vi "Положение лазера (SubVI).vi"(1 "Мишень reference":refnum<vi>, 3 "XY лазера reference":refnum<vi>, 5 "Текущ. инфо reference":refnum<vi>, 11 "error in":errorcluster, 12 "X коорд.":u16, 13 "Y коорд.":u16) -> (24 "error out":errorcluster)   [LabVIEW 2013]
doc: "Изменение положения точки текущего положения лазера и кол-ва выстрелов в точку на мишени"
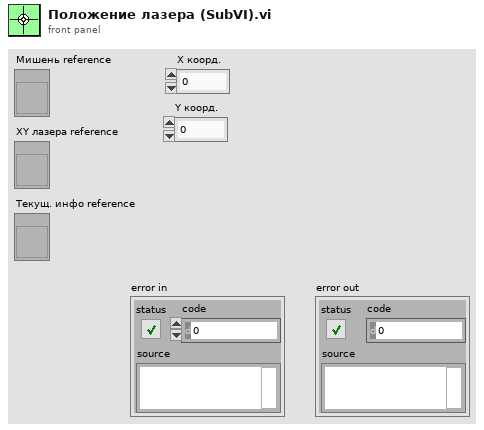
[diagram p1: front panel]
types:
  T1 = typedef "LVPositionTypeDef.ctl" = cluster{"Left":i32, "Top":i32}
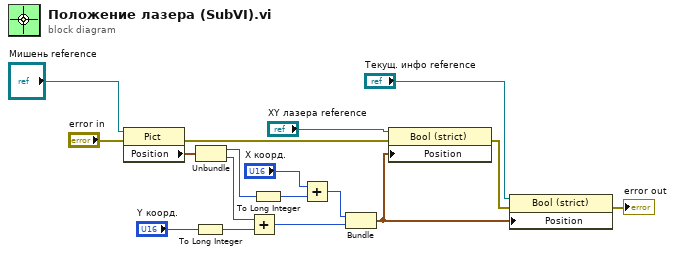
[diagram p0: block diagram]
diagram:
  n1 = property on="Property Node" class="Pict"(reference="Мишень reference", error in="error in") -> (error out=w4:errorcluster, "Position"=w5:T1)  [unwired: 1 out]
  n2 = To Long Integer(number="Y коорд.") -> (32bit integer=w12:i32)
  n3 = Unbundle(w5) -> ("Left"=w16:i32, "Top"=w8:i32)
  n4 = Add(x=w8, y=w12) -> (x+y=w7:i32)
  n5 = To Long Integer(number=w16) -> (32bit integer=w11:i32)
  n6 = Add(x="X коорд.", y=w11) -> (x+y=w6:i32)
  n7 = Bundle(w6, w7) -> (w17:cluster{i32, i32})  [unwired: 1 in]
  n8 = property on="Property Node" class="Bool (strict)"(reference="XY лазера reference", error in=w4, "Position"=w17) -> (error out=w14:errorcluster)  [unwired: 1 out]
  n9 = property on="Property Node" class="Bool (strict)"(reference="Текущ. инфо reference", error in=w14, "Position"=w17) -> (error out=→"error out":errorcluster)  [unwired: 1 out]
